vi "Measurement Config_Measure-Scope SP.vi"(8 "error in":errorcluster, 10 "Config":T1, 11 "InstruHandle":refnum<k15>) -> (0 "error out":errorcluster, 2 "Result":string)   [LabVIEW 2012]
uses:
  <instrlib>/NISCOPE/Controls/niScope scalar measurement.ctl
  <instrlib>/niScope/Measurements/niScope Multi Fetch Measurement.vi
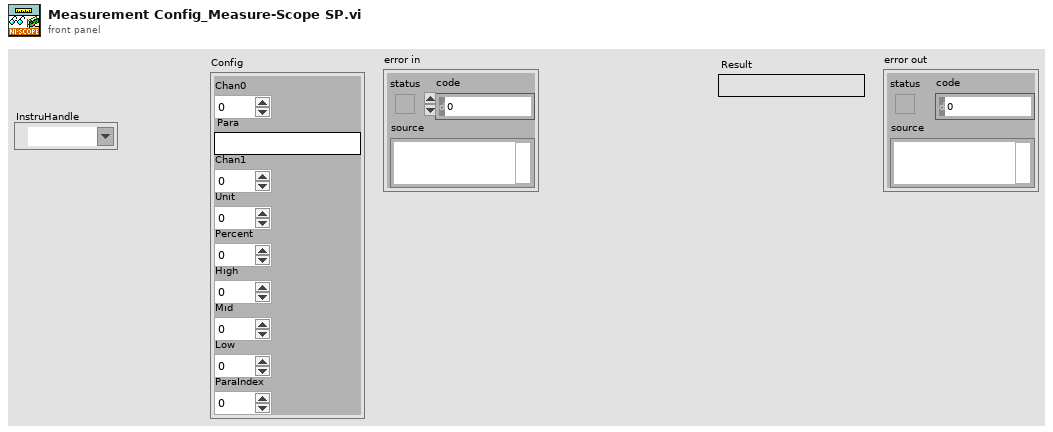
[diagram p1: front panel]
types:
  T1 = cluster{"Chan0":i32, "Para":string, "Chan1":i32, "Unit":i32, "Percent":i32, "High":dbl, "Mid":dbl, "Low":dbl, "ParaIndex":i32}
  T2 = typedef "niScope scalar measurement.ctl" = i32
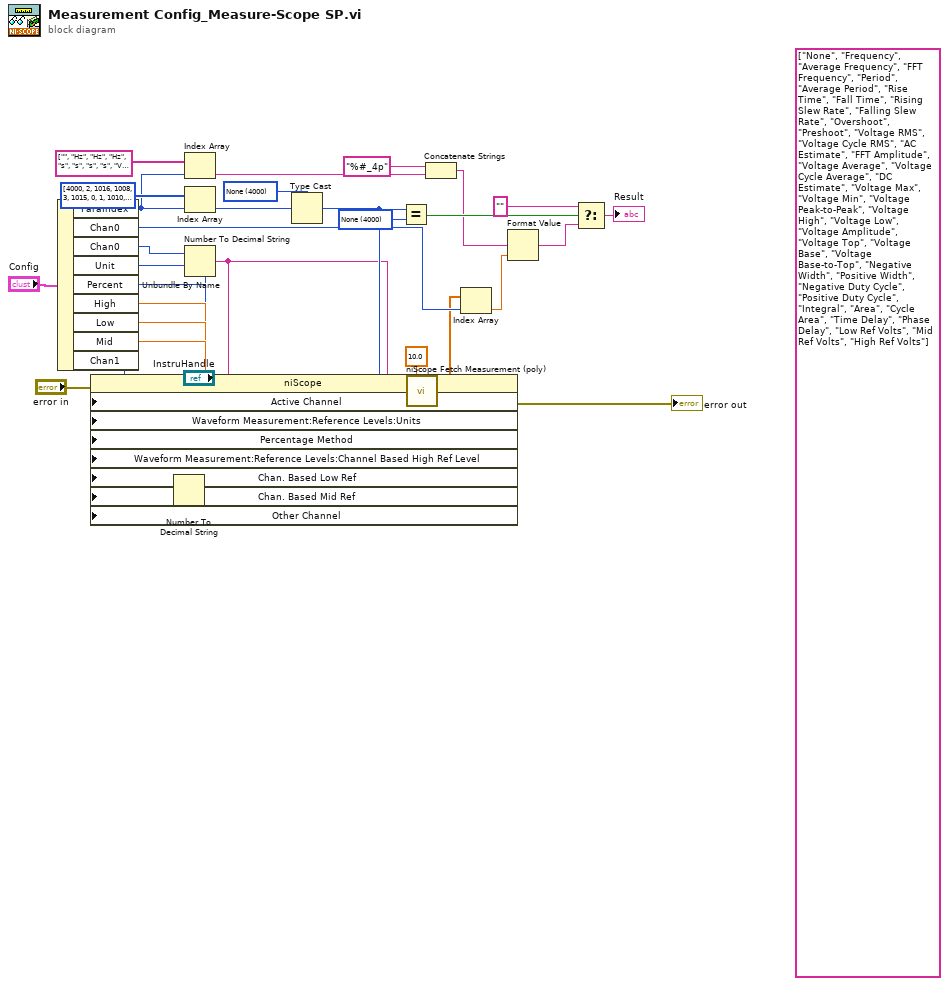
[diagram p0: block diagram]
diagram:
  (unwired) string[] ["None", "Frequency", "Average Frequency", "FFT Frequency", "Period", "Average Period", "Rise Time", "Fall Time", "Rising Slew Rate", "Falling Slew Rate", "Overshoot", "Preshoot", "Voltage RMS", "Voltage Cycle RMS", "AC Estimate", "FFT Amplitude", "Voltage Average", "Voltage Cycle Average", "DC Estimate", "Voltage Max", "Voltage Min", "Voltage Peak-to-Peak", "Voltage High", "Voltage Low", "Voltage Amplitude", "Voltage Top", "Voltage Base", "Voltage Base-to-Top", "Negative Width", "Positive Width", "Negative Duty Cycle", "Positive Duty Cycle", "Integral", "Area", "Cycle Area", "Time Delay", "Phase Delay", "Low Ref Volts", "Mid Ref Volts", "High Ref Volts"] ("数组")
  w26 = T2 4000 items=["None"=4000, "Frequency"=2, "Average Frequency"=1016, "FFT Frequency"=1008, "Period"=3, "Average Period"=1015, "Rise Time"=0, "Fall Time"=1, "Rising Slew Rate"=1010, "Falling Slew Rate"=1011, "Overshoot"=18, "Preshoot"=19, "Voltage RMS"=4, "Voltage Cycle RMS"=16, "AC Estimate"=1012, "FFT Amplitude"=1009, "Voltage Average"=10, "Voltage Cycle Average"=17, "DC Estimate"=1013, "Voltage Max"=6, "Voltage Min"=7, "Voltage Peak-to-Peak"=5, "Voltage High"=8, "Voltage Low"=9, "Voltage Amplitude"=15, "Voltage Top"=1007, "Voltage Base"=1006, "Voltage Base-to-Top"=1017, "Negative Width"=11, "Positive Width"=12, "Negative Duty Cycle"=13, "Positive Duty Cycle"=14, "Integral"=1005, "Area"=1003, "Cycle Area"=1004, "Time Delay"=1014, "Phase Delay"=1018, "Low Ref Volts"=1000, "Mid Ref Volts"=1001, "High Ref Volts"=1002, "Volt. Hist. Mean"=2000, "Volt. Hist. Stdev"=2001, "Volt. Hist. Median"=2003, "Volt. Hist. Mode"=2010, "Volt. Hist. Max"=2005, "Volt. Hist. Min"=2006, "Volt. Hist. Peak-to-Peak"=2002, "Volt. Hist. Mean + Stdev"=2007, "Volt. Hist. Mean + 2 Stdev"=2008, "Volt. Hist. Mean + 3 Stdev"=2009, "Volt. Hist. Hits"=2004, "Volt. Hist. New Hits"=2011, "Time Hist. Mean"=3000, "Time Hist. Stdev"=3001, "Time Hist. Median"=3003, "Time Hist. Mode"=3010, "Time Hist. Max"=3005, "Time Hist. Min"=3006, "Time Hist. Peak-to-Peak"=3002, "Time Hist. Mean + Stdev"=3007, "Time Hist. Mean + 2 Stdev"=3008, "Time Hist. Mean + 3 Stdev"=3009, "Time Hist. Hits"=3004, "Time Hist. New Hits"=3011] ("y")
  w22 = T2 4000 items=["None"=4000, "Frequency"=2, "Average Frequency"=1016, "FFT Frequency"=1008, "Period"=3, "Average Period"=1015, "Rise Time"=0, "Fall Time"=1, "Rising Slew Rate"=1010, "Falling Slew Rate"=1011, "Overshoot"=18, "Preshoot"=19, "Voltage RMS"=4, "Voltage Cycle RMS"=16, "AC Estimate"=1012, "FFT Amplitude"=1009, "Voltage Average"=10, "Voltage Cycle Average"=17, "DC Estimate"=1013, "Voltage Max"=6, "Voltage Min"=7, "Voltage Peak-to-Peak"=5, "Voltage High"=8, "Voltage Low"=9, "Voltage Amplitude"=15, "Voltage Top"=1007, "Voltage Base"=1006, "Voltage Base-to-Top"=1017, "Negative Width"=11, "Positive Width"=12, "Negative Duty Cycle"=13, "Positive Duty Cycle"=14, "Integral"=1005, "Area"=1003, "Cycle Area"=1004, "Time Delay"=1014, "Phase Delay"=1018, "Low Ref Volts"=1000, "Mid Ref Volts"=1001, "High Ref Volts"=1002, "Volt. Hist. Mean"=2000, "Volt. Hist. Stdev"=2001, "Volt. Hist. Median"=2003, "Volt. Hist. Mode"=2010, "Volt. Hist. Max"=2005, "Volt. Hist. Min"=2006, "Volt. Hist. Peak-to-Peak"=2002, "Volt. Hist. Mean + Stdev"=2007, "Volt. Hist. Mean + 2 Stdev"=2008, "Volt. Hist. Mean + 3 Stdev"=2009, "Volt. Hist. Hits"=2004, "Volt. Hist. New Hits"=2011, "Time Hist. Mean"=3000, "Time Hist. Stdev"=3001, "Time Hist. Median"=3003, "Time Hist. Mode"=3010, "Time Hist. Max"=3005, "Time Hist. Min"=3006, "Time Hist. Peak-to-Peak"=3002, "Time Hist. Mean + Stdev"=3007, "Time Hist. Mean + 2 Stdev"=3008, "Time Hist. Mean + 3 Stdev"=3009, "Time Hist. Hits"=3004, "Time Hist. New Hits"=3011] ("scalar measurement")
  n1 = Unbundle By Name("Config") -> ("ParaIndex"=w6:i32, "Chan0"=w31:i32, "Chan0"=w10:i32, "Unit"=w11:i32, "Percent"=w12:i32, "High"=w13:dbl, "Low"=w14:dbl, "Mid"=w15:dbl, "Chan1"=w32:i32)
  n2 = Number To Decimal String(number=w32) -> (decimal integer string=w33:string)  [unwired: 1 in]
  n3 = Index Array(array=string[] ["", "Hz", "Hz", "Hz", "s", "s", "s", "s", "V/s", "V/s", "%", "%", "VRMS", "VRMS", "VRMS", "VRMS", "V", "V", "V", "V", "V", "V", "V", "V", "V", "V", "V", "V", "s", "s", "%", "%", "V×s", "V×s", "V×s", "s", "Deg", "V", "V", "V"], index=w6) -> (element=w4:string)
  n4 = Index Array(array=i32[] [4000, 2, 1016, 1008, 3, 1015, 0, 1, 1010, 1011, 18, 19, 4, 16, 1012, 1009, 10, 17, 1013, 6, 7, 5, 8, 9, 15, 1007, 1006, 1017, 11, 12, 13, 14, 1005, 1003, 1004, 1014, 1018, 1000, 1001, 1002], index=w6) -> (element=w21:i32)
  n5 = Number To Decimal String(number=w10) -> (decimal integer string=w19:string)  [unwired: 1 in]
  n6 = property class="niScope"(reference="InstruHandle", error in="error in", "Active Channel"=w19, "Waveform Measurement:Reference Levels:Units"=w11, "Percentage Method"=w12, "Waveform Measurement:Reference Levels:Channel Based High Ref Level"=w13, "Chan. Based Low Ref"=w14, "Chan. Based Mid Ref"=w15, "Other Channel"=w33) -> (reference out=w16:refnum<k15>, error out=w17:errorcluster)
  n7 = Type Cast(type=w22, x=w21) -> (*(type *) &x=w25:T2)
  n8 = Equal?(x=w25, y=w26) -> (x = y?=w27:bool)
  n9 = call-poly <instrlib>:"niScope Fetch Measurement (poly).vi"("instrument handle"=w16, "timeout"=10.0, "channelList"=w19, "scalar measurement"=w25, "error in"=w17) -> ("results"=w24:dbl[], "error out"=→"error out":errorcluster)  [unwired: 8 in, 1 out]
  n10 = Concatenate Strings("%#_4p" ("格式字符串"), w4) -> (w3:string)
  n11 = Index Array(array=w24, index=w31) -> (element=w8:dbl)
  n12 = Format Value(format string=w3, value (0)=w8) -> (output string=w29:string)  [unwired: 1 in]
  n13 = Select(t="", s=w27, f=w29) -> (s? t:f=→"Result":string)
